vi "CameraInit.vi"(8 "error in":errorcluster, 10 "Index":i32, 11 "CameraName":string="cam0") -> (0 "error out":errorcluster, 4 "return":i32)   [LabVIEW 2019]
uses:
  [Global] CameraSessionArray.vi
  [Global] CameraNameArray.vi
  <vilib>/vision/driver/NI_Vision_Acquisition_Software.lvlib
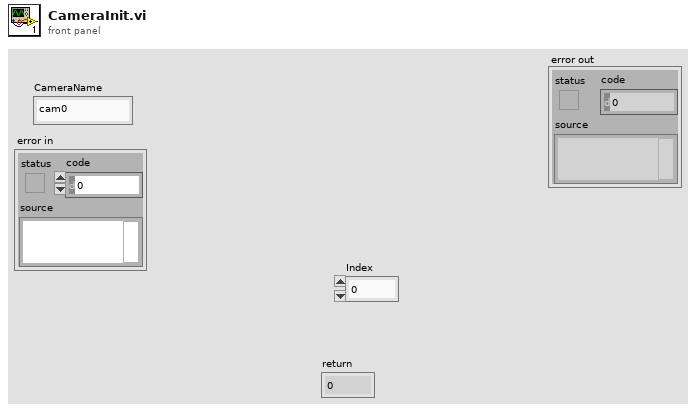
[diagram p1: front panel]
types:
  T1 = enum16{"Init", "Grab", "Get All", "Close", "Set Camera"}
  T2 = typedef "IMAQdx.ctl" = refnum<k21>
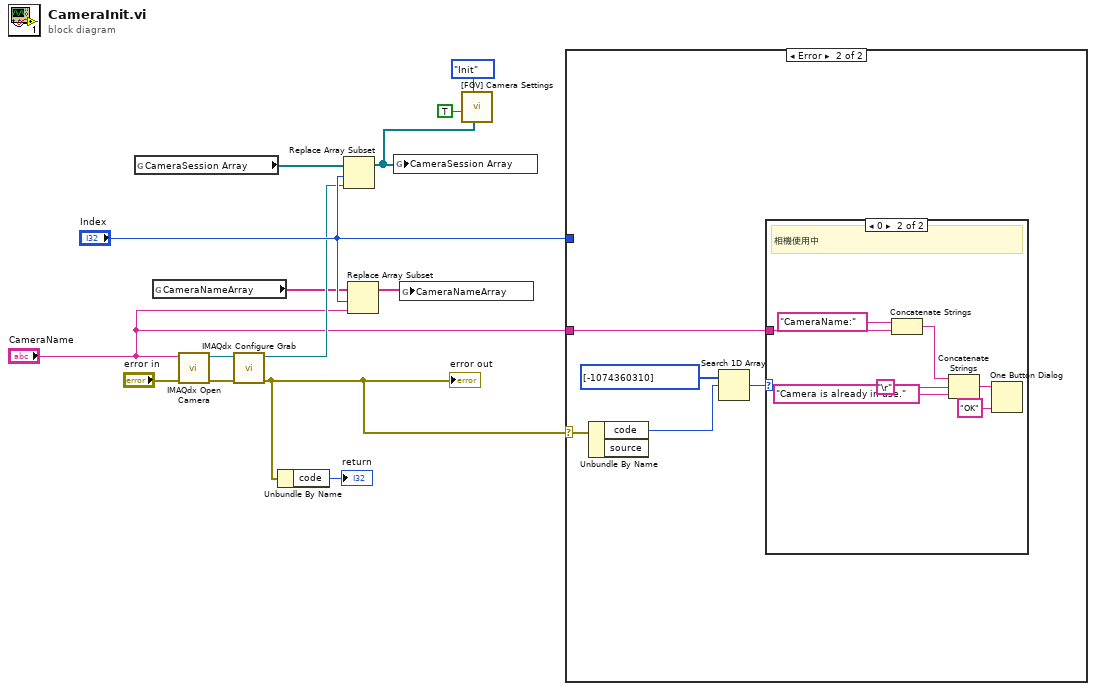
[diagram p0: block diagram]
diagram:
  n1 = global read "[Global] CameraSessionArray.vi" "CameraSession Array"() -> (w6:T2[])
  n2 = global read "[Global] CameraNameArray.vi" "CameraNameArray"() -> (w5:string[])
  n3 = call <vilib>:"IMAQdx Open Camera.vi"("error in"="error in", "Session In"="CameraName") -> ("error out"=w12:errorcluster, "Session Out"=w14:T2)  [unwired: 1 in, 7 out]
  n4 = call <vilib>:"IMAQdx Configure Grab.vi"("error in"=w12, "Session In"=w14) -> ("error out"=w10:errorcluster, "Session Out"=w8:T2)  [unwired: 8 in]
  "error out" <- w10
  n5 = Unbundle By Name(w10) -> ("code"=→"return":i32)
  n6 = Replace Array Subset(array=w6, new element=w8, index="Index") -> (w3:T2[])
  n7 = Replace Array Subset(array=w5, new element="CameraName", index="Index") -> (w7:string[])
  n8 = global write "[Global] CameraSessionArray.vi" "CameraSession Array"(w3) -> ()
  n9 = global write "[Global] CameraNameArray.vi" "CameraNameArray"(w7) -> ()
  n10 = call "[FGV] Camera Settings.vi"("CamSession"=w3, "Action"=T1."Init", "SeqOn"=TRUE) -> ()  [unwired: 6 in, 3 out]
  n11 = case shown="Error" w10 {
    selector: w10 -> [_ w19]
    tunnel: "Index" -> [_ _]
    tunnel: "CameraName" -> [_ w15]
    frame No Error {
    }
    frame Error {
      n12 = Unbundle By Name(w19) -> ("code"=w17:i32)  [unwired: 1 out]
      n13 = Search 1D Array(1D array=i32[] [-1074360310], element=w17) -> (index of element=w16:i32)  [unwired: 1 in]
      n14 = case shown="0" w16 {
        tunnel: w15 -> [_ w23]
        frame -1, Default {
        }
        frame 0 {
          # "相機使用中"
          n15 = Concatenate Strings("CameraName:", w23) -> (w20:string)
          n16 = Concatenate Strings(w20, "\r", "Camera is already in use." ("message")) -> (w24:string)
          n17 = One Button Dialog(message=w24, button name ("OK")="OK") -> ()  [unwired: 1 out]
        }
      }
    }
  }
